vi "Assign SPA values from string to axes.vi"(1 "Syntax":T1, 2 "Queried axes":string[](array[string]), 3 "Parameter no.":i32[](array[numeric]), 4 "Input string":string, 5 "error in":errorcluster, 6 "Parameter no. (hex)":u32[](array[numeric]) format="%.0x", 7 "Parameter no. format \n(Decimal: FALSE)":bool) -> (11 "Parameter no. out":i32[](array[numeric]), 12 "Queried axes out":string[](array[string]), 13 "Parameter no. (hex) out":u32[](array[numeric]) format="%.0x", 14 "Parameter values":dbl[](array[numeric]) format="%.6f", 15 "Parameter strings":string[](array[string]), 19 "error out":errorcluster)   [LabVIEW 2020]
doc: "This VI assigns numerical values / strings from input string to queried axes and hex. parameter numbers. Sub-VI for SPA?.vi."
uses:
  Syntax.ctl
panel:
  # "This vi assigns values/strings from input string to queried axes and hex. parameter numbers."
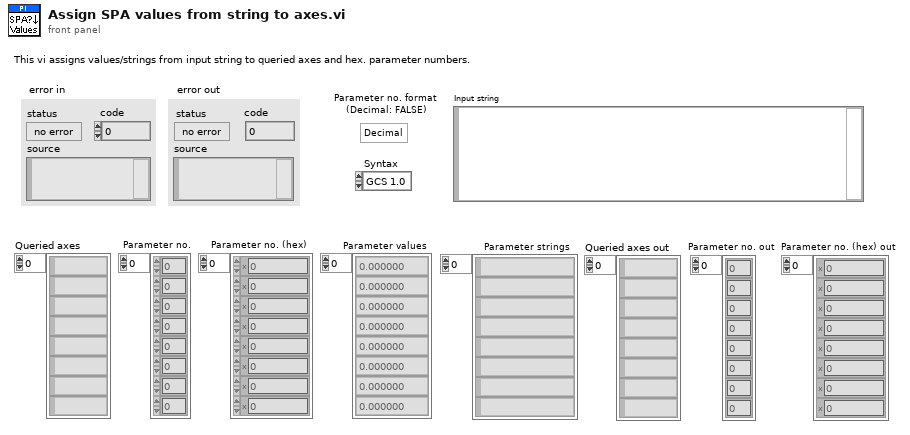
[diagram p1: front panel]
types:
  T1 = typedef "Syntax.ctl" = enum16{"GCS 1.0", "GCS 2.0", "GCS 3.0"}
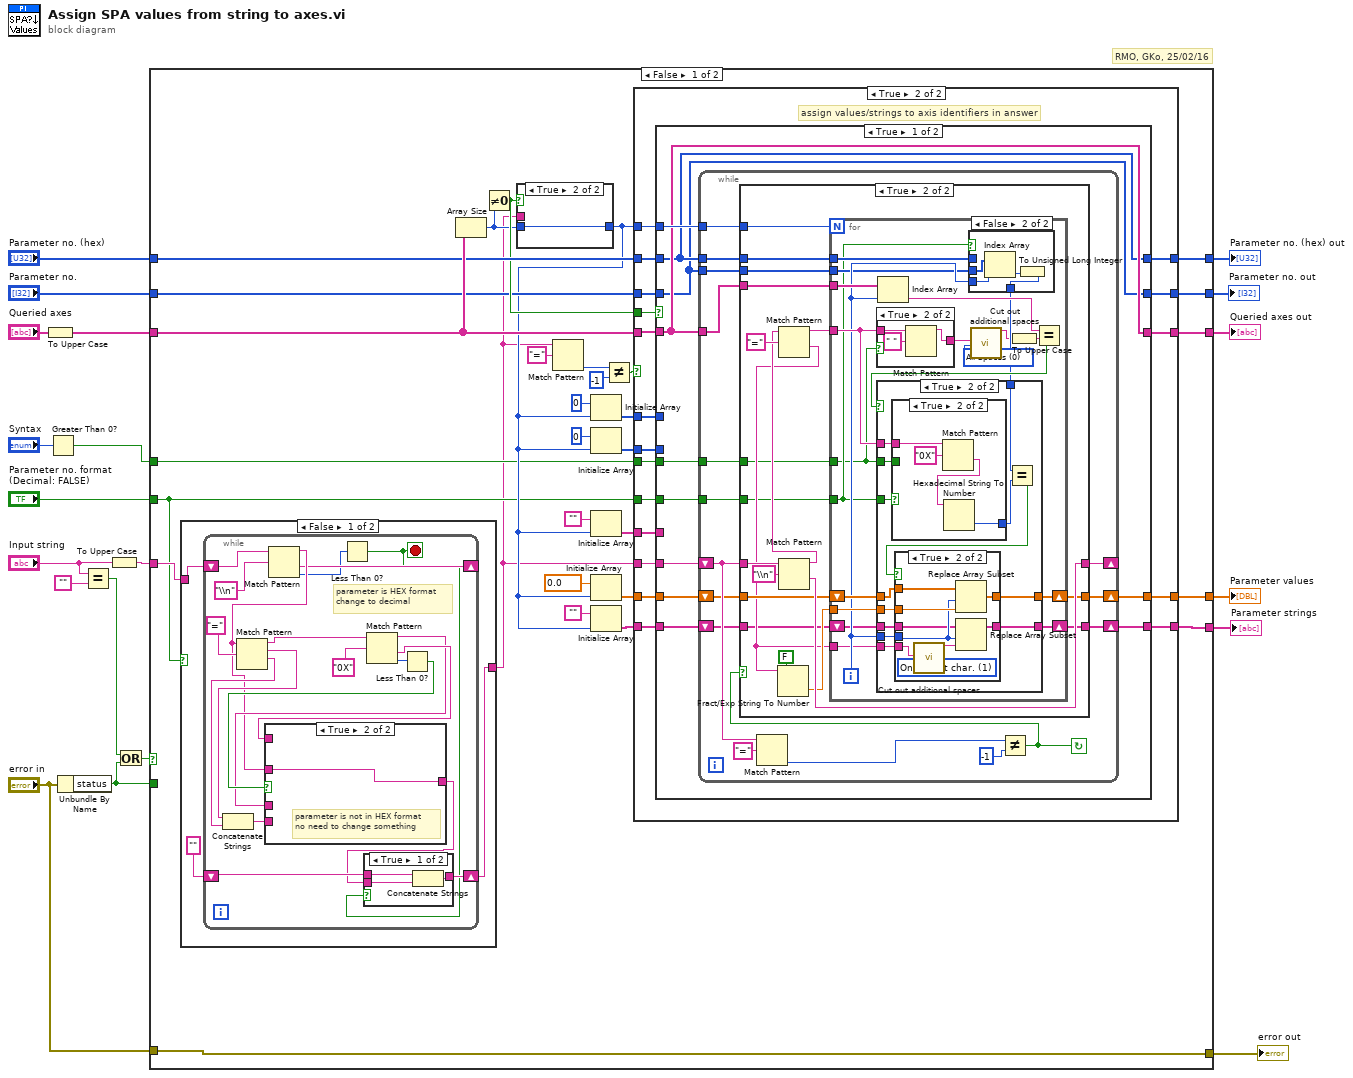
[diagram p0: block diagram]
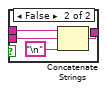
[diagram p2: hidden frame]
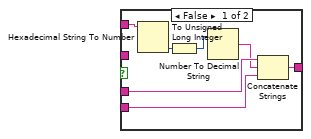
[diagram p3: hidden frame]
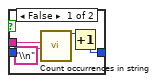
[diagram p5: hidden frame]
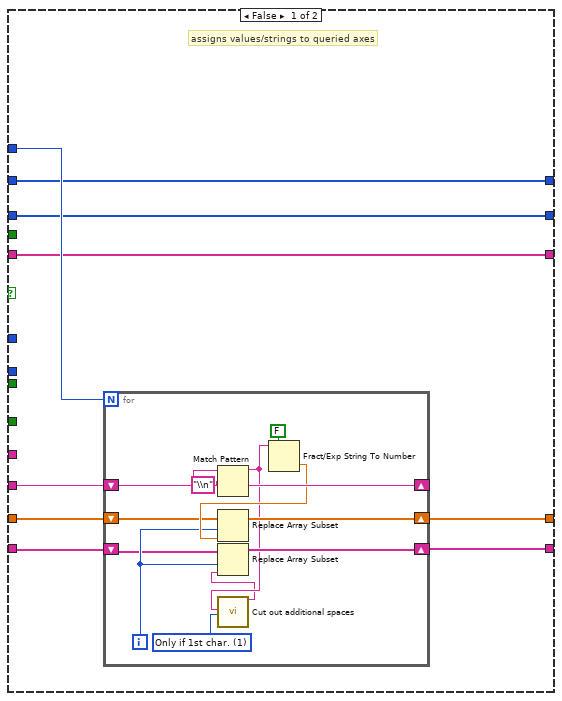
[diagram p6: hidden frame]
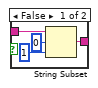
[diagram p8: hidden frame]
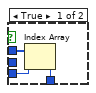
[diagram p9: hidden frame]
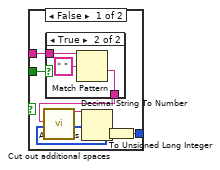
[diagram p11: hidden frame]
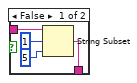
[diagram p12: hidden frame]
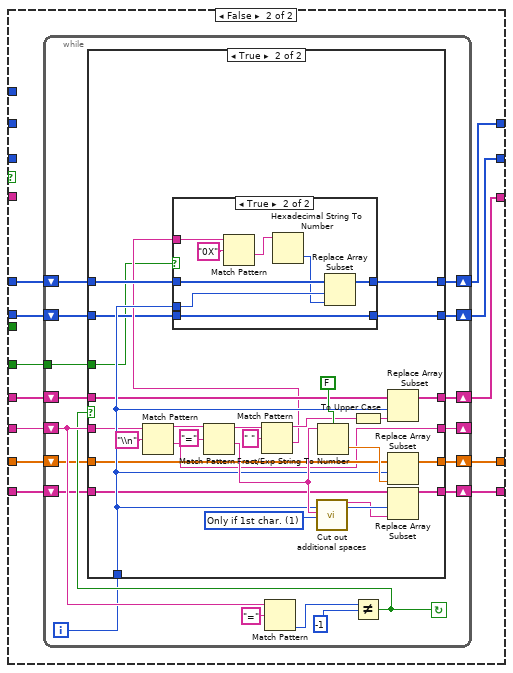
[diagram p14: hidden frame]
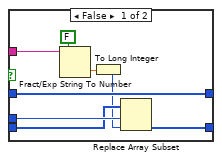
[diagram p16: hidden frame]
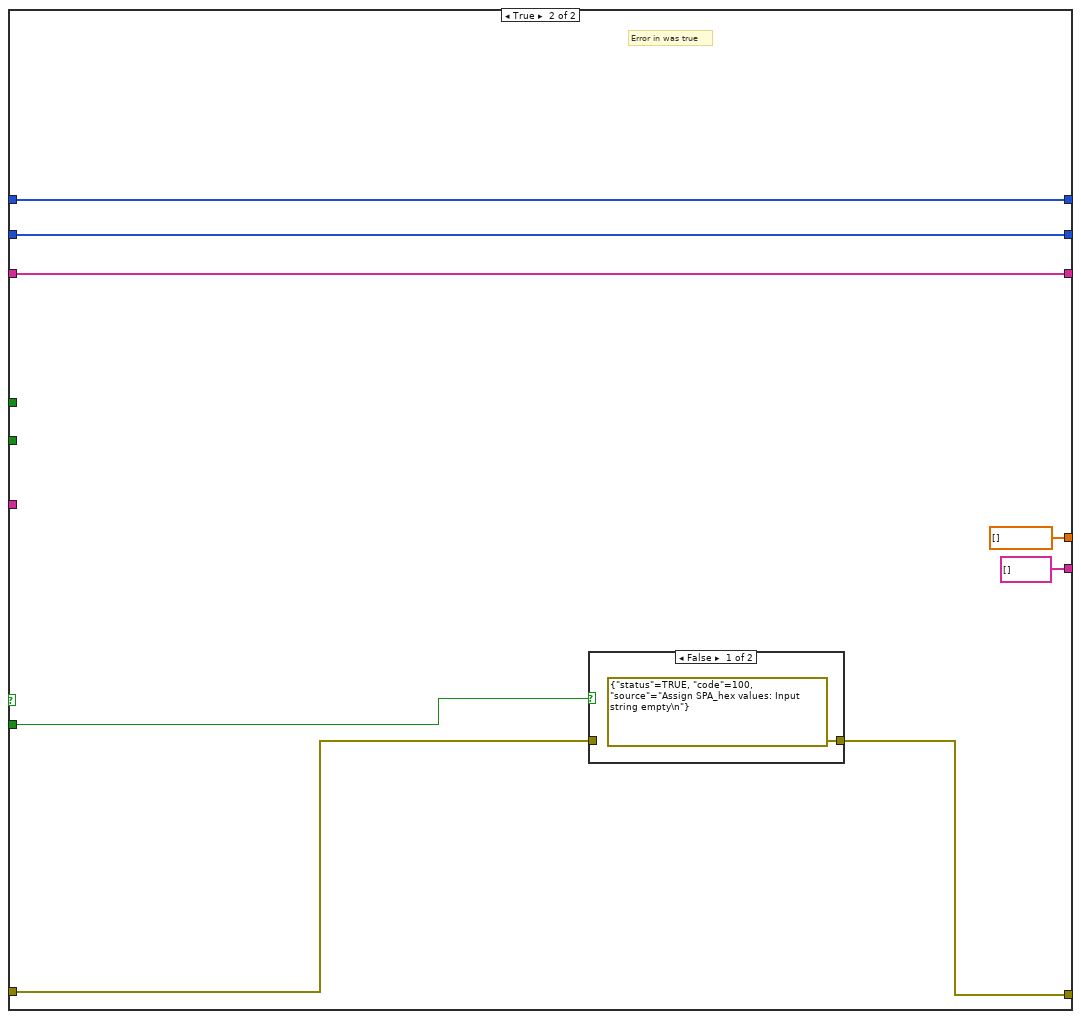
[diagram p17: hidden frame]
diagram:
  # "RMO, GKo, 25/02/16"
  n1 = To Upper Case(1:"Queried axes") -> (0:w13:string[])
  n2 = Greater Than 0?(x="Syntax") -> (x > 0?=w2:bool)
  n3 = Unbundle By Name("error in") -> ("status"=w10:bool)
  n4 = Equal?(x="Input string", y="") -> (x = y?=w11:bool)
  n5 = To Upper Case(1:"Input string") -> (0:w1:string)
  n6 = Or(x=w11, y=w10) -> (x .or. y?=w14:bool)
  n7 = case shown="False" w14 {
    tunnel: w1 -> [w23 _]
    tunnel: [w50 dbl[] [] ("Step Size")] -> w20
    tunnel: w13 -> [w49 w342]
    tunnel: [w24 w345] -> w17
    tunnel: "error in" -> [w24 w346]
    tunnel: "Parameter no. (hex)" -> [w42 w341]
    tunnel: w10 -> [_ w344]
    tunnel: [w39 string[] []] -> w9
    tunnel: [w32 w342] -> w8
    tunnel: [w31 w341] -> w7
    tunnel: "Parameter no." -> [w30 w340]
    tunnel: [w29 w340] -> w5
    tunnel: "Parameter no. format \n(Decimal: FALSE)" -> [w22 _]
    tunnel: w2 -> [w25 _]
    frame False {
      n8 = case shown="False" w22 {
        tunnel: w23 -> [w52 w88]
        tunnel: [w53 w88] -> w21
        frame False {
          n9 = while {
            shift-right: [w59] -> _
            shift-left: w52 -> [w61]
            shift-right: [w55] -> w53
            shift-left: "" -> [w57]
            stop <- w54 stop-if-true
            # "parameter is HEX format\nchange to decimal"
            n10 = Match Pattern(string=w61, regular expression="\\n") -> (before substring=w60:string, after substring=w59:string, offset past match=w58:i32)  [unwired: 2 out]
            n11 = Match Pattern(string=w60, regular expression="=") -> (before substring=w71:string, match substring=w66:string, after substring=w65:string)  [unwired: 2 out]
            n12 = Concatenate Strings(w66, w65) -> (w64:string)
            n13 = Less Than 0?(x=w58) -> (x < 0?=w54:bool)
            n14 = Match Pattern(string=w71, regular expression="0X") -> (before substring=w63:string, after substring=w67:string, offset past match=w69:i32)  [unwired: 2 out]
            n15 = Less Than 0?(x=w69) -> (x < 0?=w68:bool)
            n16 = case shown="True" w68 {
              tunnel: w60 -> [_ w87]
              tunnel: [w80 w87] -> w56
              tunnel: w67 -> [w84 _]
              tunnel: w64 -> [w81 _]
              tunnel: w63 -> [w83 _]
              frame False {
                n17 = Hexadecimal String To Number(string=w84) -> (number=w86:u32)  [unwired: 3 out]
                n18 = To Unsigned Long Integer(number=w86) -> (unsigned 32bit integer=w85:u32)
                n19 = Number To Decimal String(number=w85) -> (decimal integer string=w82:string)  [unwired: 1 out]
                n20 = Concatenate Strings(w83, w82, w81) -> (w80:string)
              }
              frame True {
                # "parameter is not in HEX format\nno need to change something"
              }
            }
            n21 = case shown="True" w54 {
              tunnel: w57 -> [w75 w79]
              tunnel: w56 -> [w74 w78]
              tunnel: [w73 w76] -> w55
              frame True {
                n22 = Concatenate Strings(w75, w74) -> (w73:string)
              }
              frame False {
                n23 = Concatenate Strings(w79, w78, "\n") -> (w76:string)
              }
            }
          }
        }
        frame True {
          # "parameter is in HEX format\nno need to change something"
        }
      }
      n24 = Array Size(array=w49) -> (size(s)=w33:i32)
      n25 = Not Equal To 0?(x=w33) -> (x != 0?=w36:bool)
      n26 = case shown="True" w36 {
        tunnel: [w89 w93] -> w27
        tunnel: w33 -> [_ w93]
        tunnel: w21 -> [w92 _]
        frame False {
          n27 = call "Count occurrences in string.vi"("Input string"=w92, "Expression"="\\n") -> ("Occurrences"=w90:i32)  [unwired: 17 out]
          n28 = Increment(x=w90) -> (x+1=w89:i32)
        }
        frame True {
        }
      }
      n29 = Match Pattern(string=w21, regular expression="=") -> (offset past match=w46:i32)  [unwired: 4 out]
      n30 = Initialize Array(u32 0 ("Element Data"), w27) -> (w34:u32[])
      n31 = Initialize Array(0 ("Element Data"), w27) -> (w26:i32[])
      n32 = Initialize Array("" ("Element Data"), w27) -> (w35:string[])
      n33 = Initialize Array(0.0 ("Element Data"), w27) -> (w43:dbl[])
      n34 = Initialize Array("" ("Element Data"), w27) -> (w40:string[])
      n35 = Not Equal?(x=w46, y=-1) -> (x != y?=w45:bool)
      n36 = case shown="True" w45 {
        tunnel: [w102 w132] -> w50
        tunnel: w21 -> [w101 w133]
        tunnel: w49 -> [w96 w131]
        tunnel: w43 -> [w100 w129]
        tunnel: w27 -> [w99 w130]
        tunnel: w42 -> [w95 w128]
        tunnel: w40 -> [w97 w127]
        tunnel: [w98 w126] -> w39
        tunnel: w36 -> [_ w125]
        tunnel: w35 -> [_ w124]
        tunnel: w34 -> [_ w123]
        tunnel: [w96 w122] -> w32
        tunnel: [w95 w121] -> w31
        tunnel: w30 -> [w94 w120]
        tunnel: [w94 w119] -> w29
        tunnel: w26 -> [_ w118]
        tunnel: w22 -> [_ w117]
        tunnel: w25 -> [_ w116]
        frame False {
          # "assigns values/strings to queried axes"
          n37 = for {
            N: w99 -> [_]
            shift-right: [w109] -> w102
            shift-left: w100 -> [w110]
            shift-right: [w114] -> _
            shift-left: w101 -> [w115]
            shift-right: [w108] -> w98
            shift-left: w97 -> [w106]
            i -> [w107]
            w103 = u16 1 items=["All Spaces", "Only if 1st char.", "Only if last char.", "Only if near \"=\""] ("Mode")
            n38 = Match Pattern(string=w115, regular expression="\\n") -> (before substring=w105:string, after substring=w114:string)  [unwired: 3 out]
            n39 = call "Cut out additional spaces.vi"("String"=w105, "Mode"=w103) -> ("String out"=w104:string)  [unwired: 17 out]
            n40 = Replace Array Subset(array=w106, new element=w104, index=w107) -> (w108:string[])
            n41 = Fract/Exp String To Number(use system decimal point (T)=FALSE, string=w105) -> (number=w111:dbl)  [unwired: 3 out]
            n42 = Replace Array Subset(array=w110, new element=w111, index=w107) -> (w109:dbl[])
          }
        }
        frame True {
          # "assign values/strings to axis identifiers in answer"
          n43 = case shown="True" w125 {
            tunnel: w133 -> [w144 w272]
            tunnel: [w143 w271] -> w132
            tunnel: w131 -> [w138 _]
            tunnel: w130 -> [w142 _]
            tunnel: w129 -> [w141 w270]
            tunnel: w128 -> [w137 _]
            tunnel: w127 -> [w140 w269]
            tunnel: [w139 w268] -> w126
            tunnel: w124 -> [_ w267]
            tunnel: w123 -> [_ w264]
            tunnel: [w138 w266] -> w122
            tunnel: [w137 w265] -> w121
            tunnel: w120 -> [w136 _]
            tunnel: [w136 w263] -> w119
            tunnel: w118 -> [_ w262]
            tunnel: w117 -> [w135 w261]
            tunnel: w116 -> [w134 _]
            frame True {
              n44 = while {
                shift-left: w140 -> [w148]
                shift-right: [w149] -> w139
                tunnel: w137 -> [w150]
                tunnel: w142 -> [w151]
                tunnel: w138 -> [w152]
                shift-left: w141 -> [w154]
                shift-right: [w153] -> w143
                shift-left: w144 -> [w157]
                shift-right: [w156] -> _
                tunnel: w136 -> [w147]
                tunnel: w135 -> [w146]
                tunnel: w134 -> [w145]
                stop <- w155 continue-if-true
                n45 = Match Pattern(string=w157, regular expression="=") -> (offset past match=w158:i32)  [unwired: 4 out]
                n46 = Not Equal?(x=w158, y=-1) -> (x != y?=w155:bool)
                n47 = case shown="True" w155 {
                  tunnel: w157 -> [w163 w181]
                  tunnel: [w163 w180] -> w156
                  tunnel: [w162 w178] -> w153
                  tunnel: w154 -> [w162 w179]
                  tunnel: w152 -> [_ w173]
                  tunnel: w151 -> [_ w170]
                  tunnel: w150 -> [_ w171]
                  tunnel: [w161 w168] -> w149
                  tunnel: w148 -> [w161 w167]
                  tunnel: w147 -> [_ w166]
                  tunnel: w146 -> [_ w165]
                  tunnel: w145 -> [_ w164]
                  frame False {
                  }
                  frame True {
                    n48 = Match Pattern(string=w181, regular expression="\\n") -> (before substring=w175:string, after substring=w180:string)  [unwired: 3 out]
                    n49 = Match Pattern(string=w175, regular expression="=") -> (before substring=w172:string, after substring=w169:string)  [unwired: 3 out]
                    n50 = Fract/Exp String To Number(use system decimal point (T)=FALSE, string=w169) -> (number=w174:dbl)  [unwired: 3 out]
                    n51 = for {
                      N: w170 -> [_]
                      tunnel: w174 -> [w202]
                      shift-right: [w200] -> w178
                      shift-left: w179 -> [w201]
                      tunnel: w173 -> [w199]
                      tunnel: w172 -> [w196]
                      tunnel: w171 -> [w195]
                      tunnel: w169 -> [w192]
                      shift-right: [w190] -> w168
                      shift-left: w167 -> [w191]
                      tunnel: w166 -> [w189]
                      tunnel: w165 -> [w188]
                      tunnel: w164 -> [w187]
                      i -> [w194]
                      w185 = u16 0 items=["All Spaces", "Only if 1st char.", "Only if last char.", "Only if near \"=\""] ("Mode")
                      n52 = case shown="True" w187 {
                        tunnel: [w204 w209] -> w186
                        tunnel: w196 -> [w203 w207]
                        frame False {
                          n53 = String Subset(string=w203, offset (0)=0, length (rest)=1 ("length")) -> (substring=w204:string)
                        }
                        frame True {
                          n54 = Match Pattern(string=w207, regular expression=" ") -> (before substring=w209:string)  [unwired: 4 out]
                        }
                      }
                      n55 = Index Array(array=w199, index=w194) -> (element=w198:string)
                      n56 = case shown="False" w188 {
                        tunnel: w195 -> [w212 _]
                        tunnel: w194 -> [w211 w216]
                        tunnel: [w210 w213] -> w193
                        tunnel: w189 -> [_ w214]
                        frame True {
                          n57 = Index Array(array=w212, index=w211) -> (element=w210:u32)
                        }
                        frame False {
                          n58 = Index Array(array=w214, index=w216) -> (element=w215:i32)
                          n59 = To Unsigned Long Integer(number=w215) -> (unsigned 32bit integer=w213:u32)
                        }
                      }
                      n60 = call "Cut out additional spaces.vi"("String"=w186, "Mode"=w185) -> ("String out"=w184:string)  [unwired: 17 out]
                      n61 = To Upper Case(1:w184) -> (0:w183:string)
                      n62 = Equal?(x=w198, y=w183) -> (x = y?=w197:bool)
                      n63 = case shown="True" w197 {
                        tunnel: w202 -> [_ w231]
                        tunnel: w194 -> [_ w228]
                        tunnel: w201 -> [w218 w230]
                        tunnel: [w218 w229] -> w200
                        tunnel: w196 -> [_ w227]
                        tunnel: w193 -> [_ w226]
                        tunnel: w192 -> [_ w223]
                        tunnel: w191 -> [w217 w222]
                        tunnel: [w217 w221] -> w190
                        tunnel: w188 -> [_ w220]
                        tunnel: w187 -> [_ w219]
                        frame False {
                        }
                        frame True {
                          n64 = case shown="True" w220 {
                            tunnel: w227 -> [w237 w249]
                            tunnel: [w232 w248] -> w225
                            tunnel: w219 -> [w236 _]
                            frame False {
                              w233 = u16 0 items=["All Spaces", "Only if 1st char.", "Only if last char.", "Only if near \"=\""] ("Mode")
                              n65 = case shown="True" w236 {
                                tunnel: [w240 w243] -> w235
                                tunnel: w237 -> [w239 w245]
                                frame False {
                                n66 = String Subset(string=w239, offset (0)=1, length (rest)=5 ("length")) -> (substring=w240:string)
                                }
                                frame True {
                                n67 = Match Pattern(string=w245, regular expression=" ") -> (after substring=w243:string)  [unwired: 4 out]
                                }
                              }
                              n68 = call "Cut out additional spaces.vi"("String"=w235, "Mode"=w233) -> ("String out"=w234:string)  [unwired: 17 out]
                              n69 = Decimal String To Number(string=w234) -> (number=w238:i32)  [unwired: 3 out]
                              n70 = To Unsigned Long Integer(number=w238) -> (unsigned 32bit integer=w232:u32)
                            }
                            frame True {
                              n71 = Match Pattern(string=w249, regular expression="0X") -> (after substring=w246:string)  [unwired: 4 out]
                              n72 = Hexadecimal String To Number(string=w246) -> (number=w248:u32)  [unwired: 3 out]
                            }
                          }
                          n73 = Equal?(x=w226, y=w225) -> (x = y?=w224:bool)
                          n74 = case shown="True" w224 {
                            tunnel: w231 -> [_ w260]
                            tunnel: w230 -> [w251 w259]
                            tunnel: [w251 w258] -> w229
                            tunnel: w228 -> [_ w257]
                            tunnel: w223 -> [_ w254]
                            tunnel: w222 -> [w250 w256]
                            tunnel: [w250 w255] -> w221
                            frame False {
                            }
                            frame True {
                              w252 = u16 1 items=["All Spaces", "Only if 1st char.", "Only if last char.", "Only if near \"=\""] ("Mode")
                              n75 = call "Cut out additional spaces.vi"("String"=w254, "Mode"=w252) -> ("String out"=w253:string)  [unwired: 17 out]
                              n76 = Replace Array Subset(array=w259, new element=w260, index=w257) -> (w258:dbl[])
                              n77 = Replace Array Subset(array=w256, new element=w253, index=w257) -> (w255:string[])
                            }
                          }
                        }
                      }
                    }
                  }
                }
              }
            }
            frame False {
              n78 = while {
                shift-left: w267 -> [w279]
                shift-right: [w276] -> w266
                shift-left: w264 -> [w278]
                shift-right: [w277] -> w265
                shift-left: w269 -> [w281]
                shift-right: [w282] -> w268
                shift-left: w270 -> [w284]
                shift-right: [w283] -> w271
                shift-left: w272 -> [w287]
                shift-right: [w286] -> _
                shift-right: [w274] -> w263
                shift-left: w262 -> [w275]
                tunnel: w261 -> [w273]
                i -> [w280]
                stop <- w285 continue-if-true
                n79 = Match Pattern(string=w287, regular expression="=") -> (offset past match=w288:i32)  [unwired: 4 out]
                n80 = Not Equal?(x=w288, y=-1) -> (x != y?=w285:bool)
                n81 = case shown="True" w285 {
                  tunnel: w287 -> [w296 w307]
                  tunnel: [w296 w306] -> w286
                  tunnel: [w295 w313] -> w283
                  tunnel: w284 -> [w295 w309]
                  tunnel: [w294 w314] -> w282
                  tunnel: w281 -> [w294 w308]
                  tunnel: w280 -> [_ w312]
                  tunnel: w279 -> [w292 w311]
                  tunnel: w278 -> [w293 w310]
                  tunnel: [w293 w305] -> w277
                  tunnel: [w292 w303] -> w276
                  tunnel: w275 -> [w291 w302]
                  tunnel: [w291 w301] -> w274
                  tunnel: w273 -> [_ w300]
                  frame False {
                  }
                  frame True {
                    w298 = u16 1 items=["All Spaces", "Only if 1st char.", "Only if last char.", "Only if near \"=\""] ("Mode")
                    n82 = Match Pattern(string=w307, regular expression="\\n") -> (before substring=w320:string, after substring=w306:string)  [unwired: 3 out]
                    n83 = Match Pattern(string=w320, regular expression="=") -> (before substring=w317:string, after substring=w318:string)  [unwired: 3 out]
                    n84 = Match Pattern(string=w317, regular expression=" ") -> (before substring=w315:string, after substring=w304:string)  [unwired: 3 out]
                    n85 = case shown="True" w300 {
                      tunnel: w312 -> [w328 w339]
                      tunnel: w310 -> [w331 w338]
                      tunnel: [w331 w337] -> w305
                      tunnel: w304 -> [w325 w335]
                      tunnel: w302 -> [w327 w332]
                      tunnel: [w326 w332] -> w301
                      frame False {
                        n86 = Fract/Exp String To Number(use system decimal point (T)=FALSE, string=w325) -> (number=w329:dbl)  [unwired: 3 out]
                        n87 = To Long Integer(number=w329) -> (32bit integer=w324:i32)
                        n88 = Replace Array Subset(array=w327, new element=w324, index=w328) -> (w326:i32[])
                      }
                      frame True {
                        n89 = Match Pattern(string=w335, regular expression="0X") -> (after substring=w334:string)  [unwired: 4 out]
                        n90 = Hexadecimal String To Number(string=w334) -> (number=w333:u32)  [unwired: 3 out]
                        n91 = Replace Array Subset(array=w338, new element=w333, index=w339) -> (w337:u32[])
                      }
                    }
                    n92 = call "Cut out additional spaces.vi"("String"=w318, "Mode"=w298) -> ("String out"=w299:string)  [unwired: 17 out]
                    n93 = Fract/Exp String To Number(use system decimal point (T)=FALSE, string=w318) -> (number=w319:dbl)  [unwired: 3 out]
                    n94 = To Upper Case(1:w315) -> (0:w297:string)
                    n95 = Replace Array Subset(array=w311, new element=w297, index=w312) -> (w303:string[])
                    n96 = Replace Array Subset(array=w309, new element=w319, index=w312) -> (w313:dbl[])
                    n97 = Replace Array Subset(array=w308, new element=w299, index=w312) -> (w314:string[])
                  }
                }
              }
            }
          }
        }
      }
    }
    frame True {
      # "Error in was true"
      n98 = case shown="False" w344 {
        tunnel: w346 -> [_ w349]
        tunnel: [errorcluster {"status"=TRUE, "code"=100, "source"="Assign SPA_hex values: Input string empty\n"} ("error out") w349] -> w345
        frame False {
        }
        frame True {
        }
      }
    }
  }
  "Parameter values" <- w20
  "error out" <- w17
  "Parameter strings" <- w9
  "Parameter no. (hex) out" <- w7
  "Queried axes out" <- w8
  "Parameter no. out" <- w5
